vi "_Sample Generator+Set freq.vi"() -> ()   [LabVIEW 2013]
panel:
  in  "TMR2 RLD value":u16
  out "VISA Refnum out":refnum<visa-resource-name>
  out "concatenated string":string
  in  "elemszam":u16
  out "error out":errorcluster
  in  "VISA resource name":refnum<visa-resource-name>
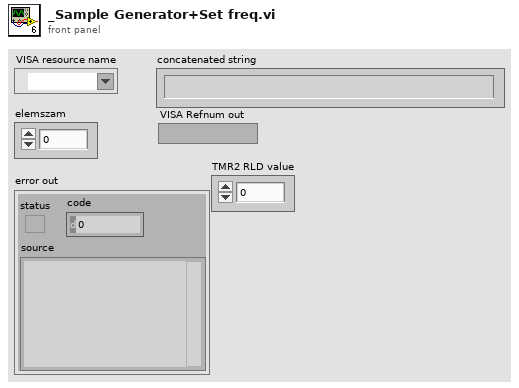
[diagram p1: front panel]
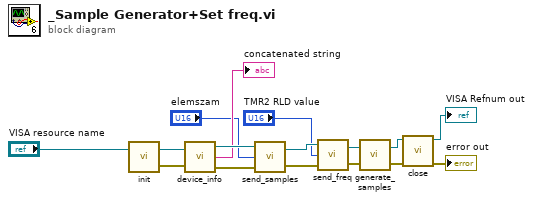
[diagram p0: block diagram]
diagram:
  n1 = call "init.vi"("VISA Refnum in"="VISA resource name") -> ("error out"=w14:errorcluster, "VISA Refnum out"=w15:refnum<visa-resource-name>)  [unwired: 1 in]
  n2 = call "device_info.vi"("VISA Refnum in"=w15, "error in (no error)"=w14) -> ("VISA Refnum out"=w13:refnum<visa-resource-name>, "concatenated string"=→"concatenated string":string, "error out"=w12:errorcluster)
  n3 = call "send_samples.vi"("error in (no error)"=w12, "elemszam"="elemszam", "VISA Refnum in"=w13) -> ("error out"=w5:errorcluster, "VISA Refnum out"=w6:refnum<visa-resource-name>)
  n4 = call "send_freq.vi"("error in (no error)"=w5, "frekvencia"="TMR2 RLD value", "VISA Refnum in"=w6) -> ("error out"=w3:errorcluster, "VISA Refnum out"=w4:refnum<visa-resource-name>)
  n5 = call "generate_samples.vi"("error in (no error)"=w3, "VISA Refnum in"=w4) -> ("error out"=w7:errorcluster, "VISA Refnum out"=w8:refnum<visa-resource-name>)
  n6 = call "close.vi"("error in (no error)"=w7, "VISA resource name"=w8) -> ("error out"=→"error out":errorcluster, "VISA resource name out"=→"VISA Refnum out":refnum<visa-resource-name>)  [unwired: 4 in]
